vi "HIOKI PW3390 Acquisition Wave+Noise.vi"() -> ()   [LabVIEW 2009]
doc: "Outputs the voltage and current waveforms of the specified channel and noise measurement data."
uses:
  <instrlib>/PW3390/Common/_Initialize/HIOKI PW3390 Initialize LAN.vi
panel:
  out "error out":errorcluster
  in  "Window Type (1: Hanning)":enum16{"rectangular", "hanning", "flat top"}(ring)=enum."hanning"
  in  "Lowest Noise Freq (1: 1kHz)":T1(ring)=enum."1kHz"
  in  "Points (2: 10000)":enum16{"1000", "5000", "10000", "50000"}(ring)=enum."10000"
  in  "Sampling (4: 250kS/s)":T2(ring)=enum."250kS"
  out "A out":dbl[](array[numeric]) format="%.2e"
  out "Af out":dbl[](array[numeric]) format="%.2f"
  out "V out":dbl[](array[numeric]) format="%.2e"
  out "Vf out":dbl[](array[numeric]) format="%.2f"
  in  "Analysis CH":enum16{"CH1", "CH2", "CH3", "CH4"}(ring)
  out "I Wave":waveform(sgl)(graph)
  out "U Wave":waveform(sgl)(graph)
  in  "IP Address":string="192.168.1.1"
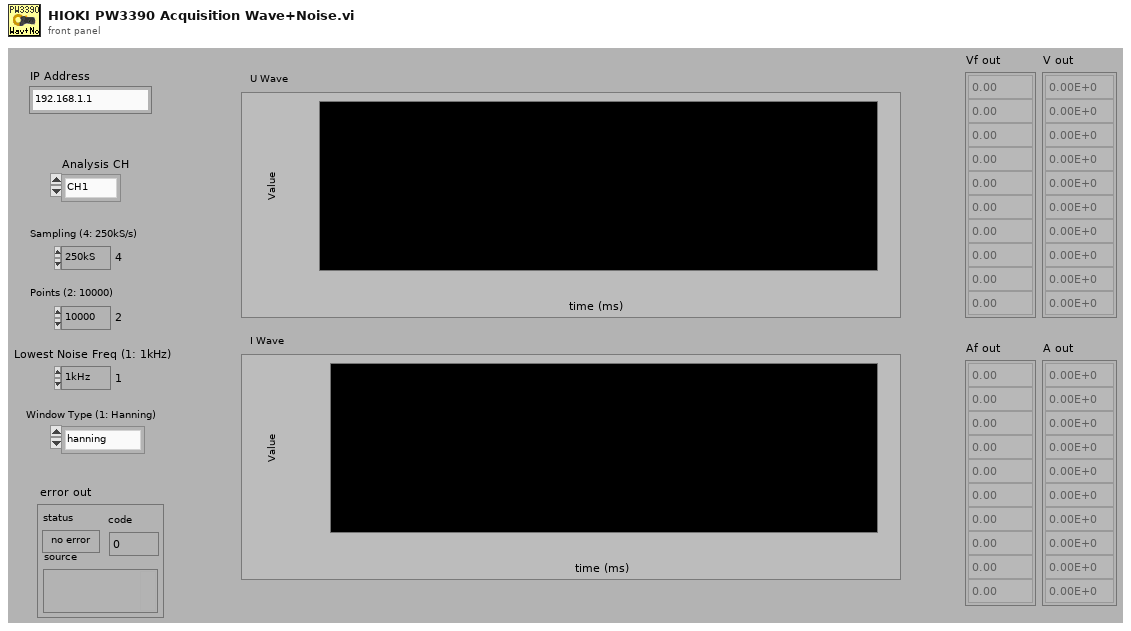
[diagram p1: front panel]
types:
  T1 = enum16{"OFF", "1kHz", "2kHz", "3kHz", "4kHz", "5kHz", "6kHz", "7kHz", "8kHz", "9kHz", "10kHz"}
  T2 = enum16{"10kS", "25kS", "50kS", "100kS", "250kS", "500kS"}
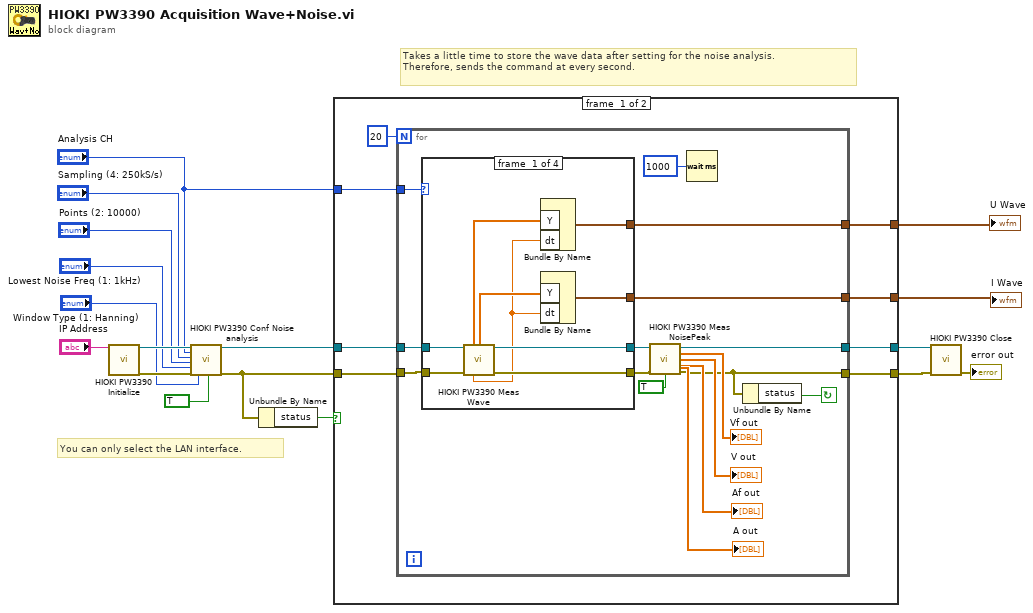
[diagram p0: block diagram]
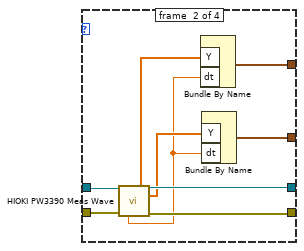
[diagram p2: hidden frame]
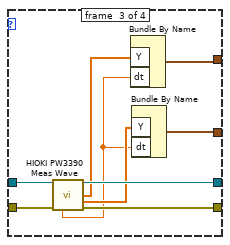
[diagram p3: hidden frame]
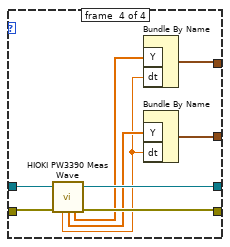
[diagram p4: hidden frame]
diagram:
  # "Takes a little time to store the wave data after setting for the noise analysis.\nTherefore, sends the command at every second."
  # "You can only select the LAN interface."
  n1 = call-poly <instrlib>:"HIOKI PW3390 Initialize.vi"("IP Address"="IP Address") -> ("VISA Resource out"=w13:refnum<visa-resource-name>, "error out"=w14:errorcluster)  [unwired: 12 in, 1 out]
  n2 = call <instrlib>:"HIOKI PW3390 Conf Noise analysis.vi"("VISA Resource"=w13, "Analysis CH (0: CH1)"="Analysis CH", "Sampling (4: 250kS)"="Sampling (4: 250kS/s)", "Points (2: 10000)"="Points (2: 10000)", "Lowest Noise Freq (1: 1kHz)"="Lowest Noise Freq (1: 1kHz)", "error in (no error)"=w14, "Window Type (1: Hanning)"="Window Type (1: Hanning)", "Error Out (F: Off)"=TRUE) -> ("VISA Resource out"=w4:refnum<visa-resource-name>, "error out"=w1:errorcluster)  [unwired: 5 in, 5 out]
  n3 = Unbundle By Name(w1) -> ("status"=w2:bool)
  n4 = case shown="FALSE" w2 {
    tunnel: [w25 _] -> w16
    tunnel: [w24 _] -> w15
    tunnel: "Analysis CH" -> [w23 _]
    tunnel: [w22 w79] -> w11
    tunnel: [w21 w78] -> w10
    tunnel: w4 -> [w19 w79]
    tunnel: w1 -> [w18 w78]
    frame #0 {
      n5 = for {
        N: 20 -> [_]
        tunnel: [w41] -> w25
        tunnel: [w40] -> w24
        tunnel: w19 -> [w39]
        tunnel: w18 -> [w38]
        tunnel: w23 -> [w37]
        tunnel: [w28] -> w22
        tunnel: [w26] -> w21
        stop <- w36 continue-if-true
        n6 = case shown="\"CH1\"" w37 {
          tunnel: [w50 w59 w68 w77] -> w41
          tunnel: [w49 w58 w67 w76] -> w40
          tunnel: [w48 w56 w66 w74] -> w30
          tunnel: [w47 w57 w65 w75] -> w29
          tunnel: w39 -> [w43 w52 w61 w70]
          tunnel: w38 -> [w42 w51 w60 w69]
          frame #0 {
            n7 = call <instrlib>:"HIOKI PW3390 Meas Wave.vi"("VISA Resource"=w43, "error in (no error)"=w42) -> ("U1 Value out"=w46:sgl[], "I1 Value out"=w45:sgl[], "VISA Resource out"=w48:refnum<visa-resource-name>, "dt out"=w44:dbl, "error out"=w47:errorcluster)  [unwired: 3 in, 6 out]
            n8 = Bundle By Name("Y"=w46, "dt"=w44) -> (w50:waveform(sgl))  [unwired: 1 in]
            n9 = Bundle By Name("Y"=w45, "dt"=w44) -> (w49:waveform(sgl))  [unwired: 1 in]
          }
          frame #1 {
            n10 = call <instrlib>:"HIOKI PW3390 Meas Wave.vi"("VISA Resource"=w52, "error in (no error)"=w51) -> ("U2 Value out"=w54:sgl[], "VISA Resource out"=w56:refnum<visa-resource-name>, "I2 Value out"=w55:sgl[], "dt out"=w53:dbl, "error out"=w57:errorcluster)  [unwired: 3 in, 6 out]
            n11 = Bundle By Name("Y"=w54, "dt"=w53) -> (w59:waveform(sgl))  [unwired: 1 in]
            n12 = Bundle By Name("Y"=w55, "dt"=w53) -> (w58:waveform(sgl))  [unwired: 1 in]
          }
          frame #2 {
            n13 = call <instrlib>:"HIOKI PW3390 Meas Wave.vi"("VISA Resource"=w61, "error in (no error)"=w60) -> ("VISA Resource out"=w66:refnum<visa-resource-name>, "U3 Value out"=w64:sgl[], "I3 Value out"=w63:sgl[], "dt out"=w62:dbl, "error out"=w65:errorcluster)  [unwired: 3 in, 6 out]
            n14 = Bundle By Name("Y"=w64, "dt"=w62) -> (w68:waveform(sgl))  [unwired: 1 in]
            n15 = Bundle By Name("Y"=w63, "dt"=w62) -> (w67:waveform(sgl))  [unwired: 1 in]
          }
          frame #3 {
            n16 = call <instrlib>:"HIOKI PW3390 Meas Wave.vi"("VISA Resource"=w70, "error in (no error)"=w69) -> ("VISA Resource out"=w74:refnum<visa-resource-name>, "dt out"=w71:dbl, "I4 Value out"=w72:sgl[], "U4 Value out"=w73:sgl[], "error out"=w75:errorcluster)  [unwired: 3 in, 6 out]
            n17 = Bundle By Name("Y"=w73, "dt"=w71) -> (w77:waveform(sgl))  [unwired: 1 in]
            n18 = Bundle By Name("Y"=w72, "dt"=w71) -> (w76:waveform(sgl))  [unwired: 1 in]
          }
        }
        n19 = call <instrlib>:"HIOKI PW3390 Meas NoisePeak.vi"("VISA Resource"=w30, "error in (no error)"=w29, "Error Out (F: Off)"=TRUE) -> ("VISA Resource out"=w28:refnum<visa-resource-name>, "Vf out"=→"Vf out":dbl[], "V out"=→"V out":dbl[], "Af out"=→"Af out":dbl[], "A out"=→"A out":dbl[], "error out"=w26:errorcluster)  [unwired: 7 in]
        n20 = Wait (ms)(milliseconds to wait=u32 1000 ("ミリ秒待機時間")) -> ()  [unwired: 1 out]
        n21 = Unbundle By Name(w26) -> ("status"=w36:bool)
      }
    }
    frame #1 {
    }
  }
  "U Wave" <- w16
  "I Wave" <- w15
  n22 = call <instrlib>:"HIOKI PW3390 Close.vi"("VISA Resource"=w11, "error in (no error)"=w10) -> ("error out"=→"error out":errorcluster)  [unwired: 13 in]
